vi "Build_Device_Details.vi"(8 "Audio Settings":T1, 11 "Audio Device Details":T2(array[cluster])) -> (0 "Sampling Frequncy Hz":dbl, 1 "Depth":i32, 2 "Channel":i32, 3 "Device ID":u32, 4 "minFreq":dbl, 5 "maxFreq":dbl)   [LabVIEW 2020]
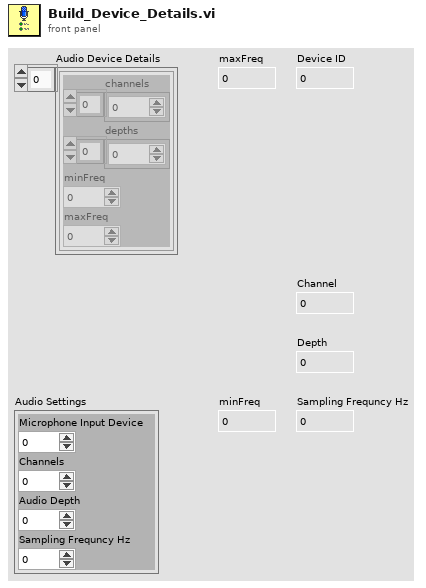
[diagram p1: front panel]
types:
  T1 = cluster{"Microphone Input Device":u32, "Channels":i32, "Audio Depth":i32, "Sampling Frequncy Hz":dbl}
  T2 = cluster{"channels":i32[], "depths":i32[], "minFreq":dbl, "maxFreq":dbl}[]
  T3 = cluster{"channels":i32[], "depths":i32[], "minFreq":dbl, "maxFreq":dbl}
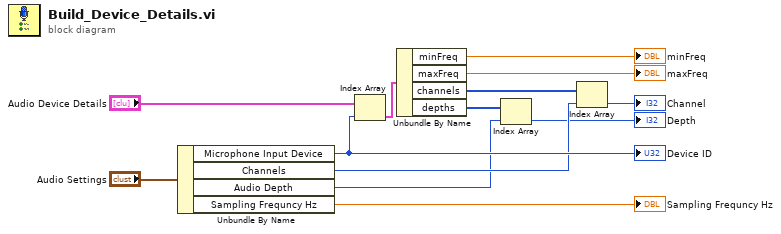
[diagram p0: block diagram]
diagram:
  n1 = Unbundle By Name("Audio Settings") -> ("Microphone Input Device"=w13:u32, "Channels"=w7:i32, "Audio Depth"=w6:i32, "Sampling Frequncy Hz"=→"Sampling Frequncy Hz":dbl)
  "Device ID" <- w13
  n2 = Index Array(array="Audio Device Details", index=w13) -> (element=w10:T3)
  n3 = Unbundle By Name(w10) -> ("minFreq"=→"minFreq":dbl, "maxFreq"=→"maxFreq":dbl, "channels"=w9:i32[], "depths"=w8:i32[])
  n4 = Index Array(array=w8, index=w6) -> (element=→"Depth":i32)
  n5 = Index Array(array=w9, index=w7) -> (element=→"Channel":i32)
